vi "Get Read Out Time.vi"(8 "error in (no error)":errorcluster, 11 "ReadOutTime":sgl) -> (0 "error out":errorcluster, 2 "function return":u32, 3 "ReadOutTime out":sgl)   [LabVIEW 2014, in "atmcd32d.lvlib"]
doc: "unsigned int WINAPI GetReadOutTime(float * ReadOutTime);"
uses:
  atmcd32d.lvlib
  atmcd32d.dll
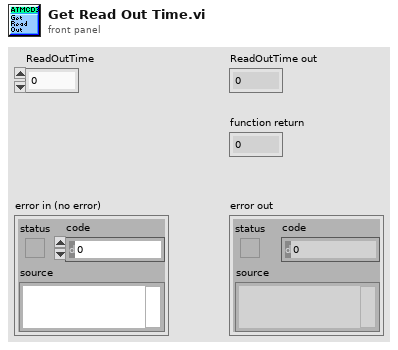
[diagram p1: front panel]
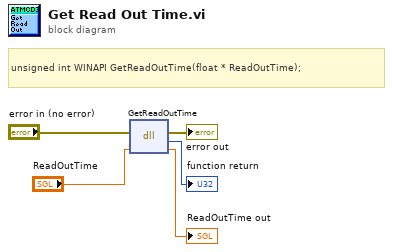
[diagram p0: block diagram]
diagram:
  # "unsigned int WINAPI GetReadOutTime(float * ReadOutTime);"
  n1 = dll-call lib="C:/Users/Bakir/Documents/Lambda2-Testing/lib/Andorlib/atmcd32d.*" fn="GetReadOutTime"(error in="error in (no error)", "ReadOutTime"="ReadOutTime") -> (error out=→"error out":errorcluster, →"function return":u32, "ReadOutTime"=→"ReadOutTime out":sgl)  [unwired: 2 in, 1 out]
